vi "Populate Complete List Items.vi"(1 "List":string) -> (0 "Complete List Items":string[](array[string]))   [LabVIEW 2020, in "AoC 2022.lvlib"]
uses:
  AoC 2022.lvlib
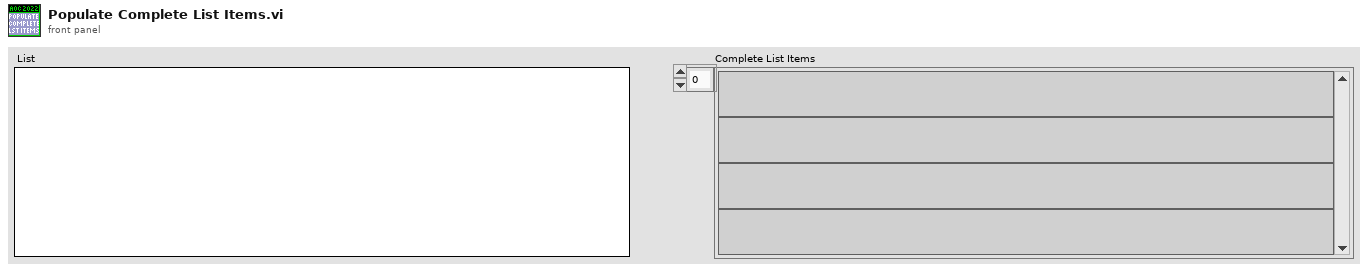
[diagram p1: front panel]
types:
  T1 = typedef "AoC 2022.lvlib/Item.ctl" = cluster{"Item Type":T2, "Item":string}
  T2 = typedef "AoC 2022.lvlib/Item Type.ctl" = enum16{"Integer", "List"}
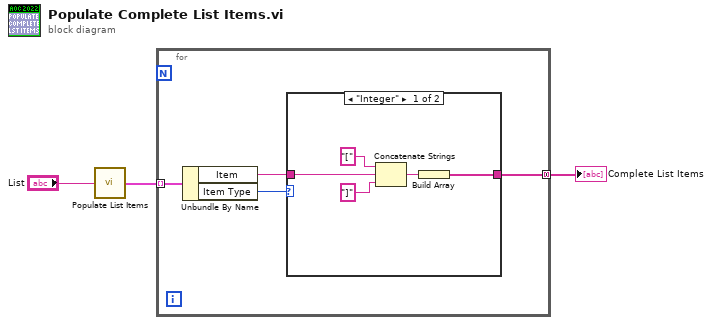
[diagram p0: block diagram]
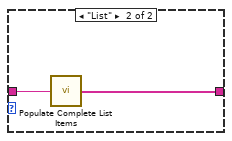
[diagram p2: hidden frame]
diagram:
  n1 = call "Populate List Items.vi"("List"="List") -> ("Items"=w2:T1[])
  n2 = for {
    tunnel: w2 -> [w7] mode=indexing
    tunnel: [w4] -> w3 mode=concatenating
    n3 = Unbundle By Name(w7) -> ("Item"=w6:string, "Item Type"=w5:T2)
    n4 = case shown="\"Integer\"" w5 {
      tunnel: w6 -> [w11 w14]
      tunnel: [w8 w13] -> w4
      frame "Integer" {
        n5 = Concatenate Strings("[", w11, "]") -> (w9:string)
        n6 = Build Array(w9) -> (w8:string[])
      }
      frame "List" {
        n7 = call "Populate Complete List Items.vi"("List"=w14) -> ("Complete List Items"=w13:string[])
      }
    }
  }
  "Complete List Items" <- w3
